vi "New Root.vi"(8 "error in (no error)":errorcluster) -> (0 "error out":errorcluster, 2 "normal log":refnum<class "Normal Log.lvclass">)   [LabVIEW 2020, in "Normal Log.lvlib" / "Normal Log.lvclass"]
uses:
  Normal Log.lvclass
  <vilib>/ActorFramework/Actor/Actor.lvclass
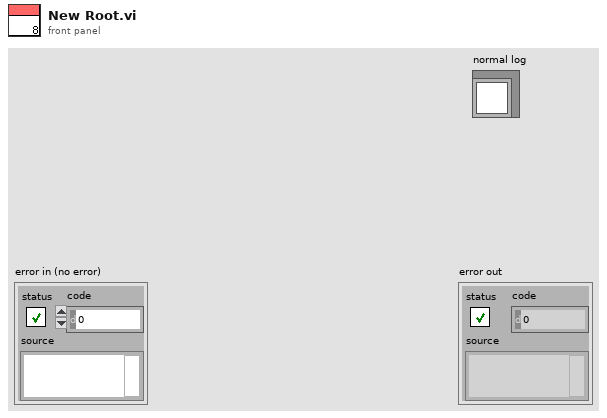
[diagram p1: front panel]
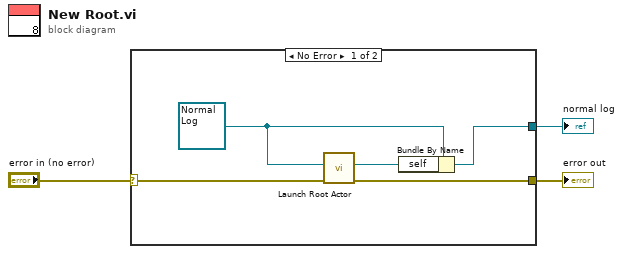
[diagram p0: block diagram]
diagram:
  n1 = case shown="No Error" "error in (no error)" {
    selector: "error in (no error)" -> [w8 w9]
    tunnel: [w5 w9] -> w2
    tunnel: [w6 _] -> w1
    frame No Error {
      w4 = refnum<class "Normal Log.lvclass"> refnum ("Normal Log in")
      n2 = call <vilib>:"Launch Root Actor.vi"("error in (no error)"=w8, "Actor"=w4) -> ("error out"=w5:errorcluster, "Actor's Enqueuer"=w7:refnum<class "Message Enqueuer.lvclass">)  [unwired: 8 in]
      n3 = Bundle By Name(cluster=w4, "self"=w7) -> (w6:refnum<class "Normal Log.lvclass">)
    }
    frame Error {
    }
  }
  "error out" <- w2
  "normal log" <- w1
